vi "brake.vi"(8 "Error In":errorcluster, 9 "write":bool, 11 "Enum":enum16{"read", "write"}(ring)) -> (0 "Error Out":errorcluster, 1 "read":bool)   [LabVIEW 2019]
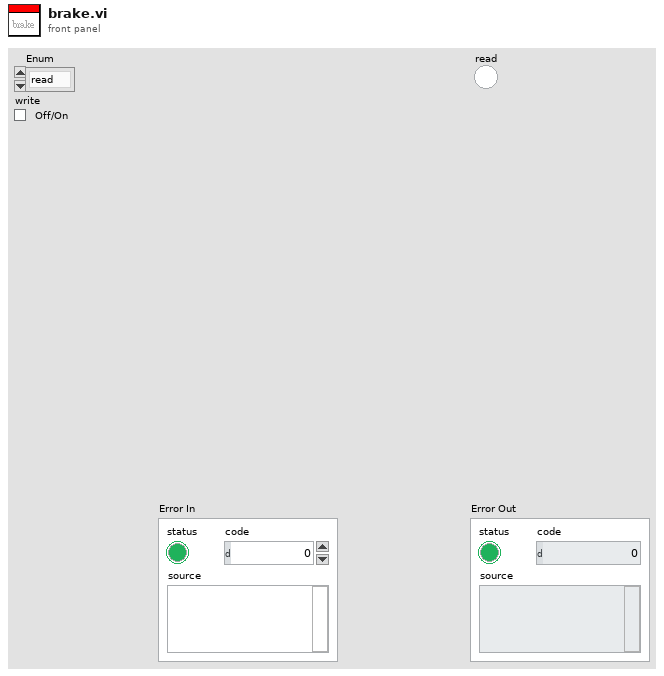
[diagram p1: front panel]
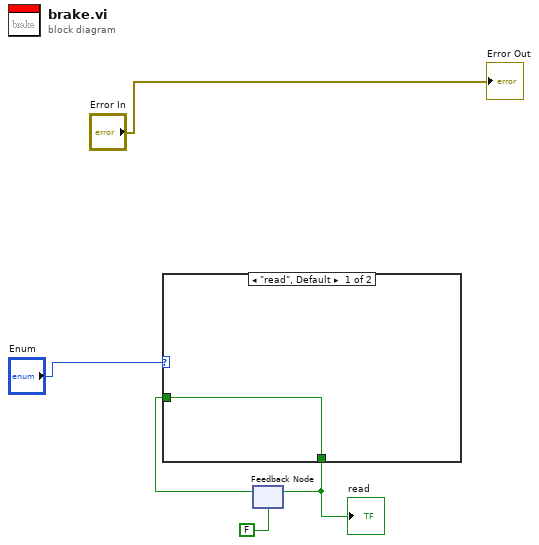
[diagram p0: block diagram]
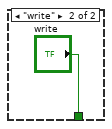
[diagram p2: hidden frame]
diagram:
  n1 = feedback #1(FALSE) -> (w3:bool)
  n2 = case shown="\"read\", Default" "Enum" {
    tunnel: w3 -> [w6 _]
    tunnel: [w6 "write"] -> w2
    frame "read", Default {
    }
    frame "write" {
    }
  }
  "read" <- w2
  n3 = feedback-in #1(w2) -> ()
  "Error Out" <- "Error In"
